vi "Current.vi"(9 "Maximum Current (pA)":dbl, 10 "Setpoint Current (A)":dbl, 11 "Current (A)":dbl) -> (1 "Current Maxed?":bool, 2 "Raw Current (pA)":dbl, 3 "Filtered Current (pA)":dbl)   [LabVIEW 2019]
uses:
  <vilib>/Analysis/3filter.llb/Filter Passband Type.ctl
  <userlib>/HapticSTM/HapticSTM.lvlib
  <vilib>/ptbypt/NI_PtbyPt.lvlib
  <vilib>/Analysis/NI_AALBase.lvlib
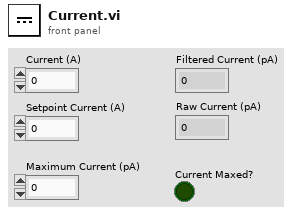
[diagram p1: front panel]
types:
  T1 = typedef "NI_AALBase.lvlib/Filter Passband Type.ctl" = enum32{"Lowpass", "Highpass", "Bandpass", "Bandstop"}
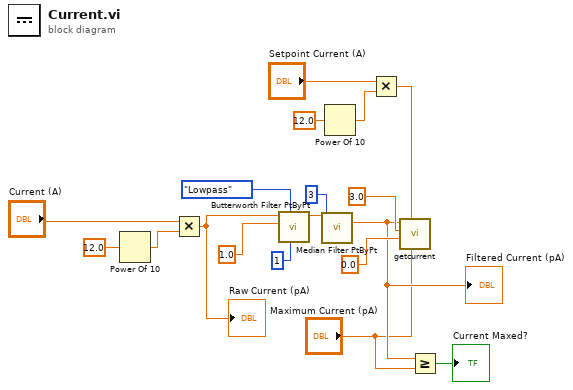
[diagram p0: block diagram]
diagram:
  n1 = Power Of 10(x=12.0) -> (10^x=w6:dbl)
  n2 = Multiply(x="Current (A)", y=w6) -> (x*y=w4:dbl)
  "Raw Current (pA)" <- w4
  n3 = call <vilib>:"Butterworth Filter PtByPt.vi"("order"=1, "filter type"=Filter_Passband_Type."Lowpass", "sampling freq: fs"=1.0, "x"=w4) -> ("Filtered x"=w13:dbl)  [unwired: 5 in, 1 out]
  n4 = call <vilib>:"Median Filter PtByPt.vi"("rank"=3, "x"=w13) -> ("Filtered x"=w3:dbl)  [unwired: 2 in, 1 out]
  "Filtered Current (pA)" <- w3
  n5 = Power Of 10(x=12.0) -> (10^x=w11:dbl)
  n6 = Multiply(x="Setpoint Current (A)", y=w11) -> (x*y=w8:dbl)
  n7 = call <userlib>:"getcurrent.vi"("maxcurrentin"="Maximum Current (pA)", "setpoint"=w8, "minforcey"=0.0, "maxforcey"=3.0, "currentin"=w3) -> ()  [unwired: 7 in]
  n8 = Greater Or Equal?(x=w3, y="Maximum Current (pA)") -> (x >= y?=→"Current Maxed?":bool)
